vi "Pre Launch Init.vi"(11 "Nested in":refnum<class "ENG Actor.lvclass">) -> (0 "error out":errorcluster, 3 "Nested out":refnum<class "ENG Actor.lvclass">)   [LabVIEW 2020, in "ENG Actor.lvlib" / "ENG Actor.lvclass"]
doc: "(<B>Filename</B>: Actor Framework.lvlib:Actor.lvclass:Pre Launch Init.vi)\n\nDefines behavior that occurs after the Launch Nested Actor method is invoked but before the actor's Actor Core method begins running.\n\nBy default, this method does nothing. A descendant class may override it to define behavior."
uses:
  ENG Actor.lvclass
  C:/Program Files (x86)/National Instruments/LabVIEW 2020/vi.lib/ActorFramework/Actor/Actor.lvclass
  ENG Actor.lvclass/ENG Actor.ctl
  <vilib>/ActorFramework/Actor/Actor.lvclass/Actor.ctl
  <vilib>/ActorFramework/Message Enqueuer/Message Enqueuer.lvclass/Message Enqueuer.ctl
  <vilib>/ActorFramework/Message Enqueuer/Init from Existing Queue.vi
  <vilib>/ActorFramework/Message Enqueuer/Enqueue.vi
  ENG Actor Messages/Init Msg/Init Msg.lvclass
  C:/Program Files (x86)/National Instruments/LabVIEW 2020/vi.lib/ActorFramework/Message/Message.lvclass
  <vilib>/ActorFramework/Message Priority Queue/Priority Enqueue.vi
  <vilib>/ActorFramework/Message Enqueuer/Message Enqueuer.lvclass
  <vilib>/ActorFramework/Actor/Actor.lvclass
  ENG Actor Messages/Update MSG Msg/Update MSG Msg.lvclass
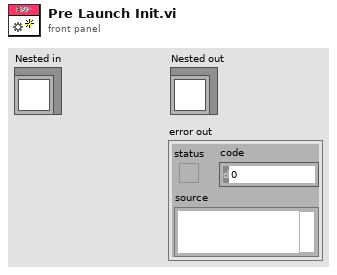
[diagram p1: front panel]
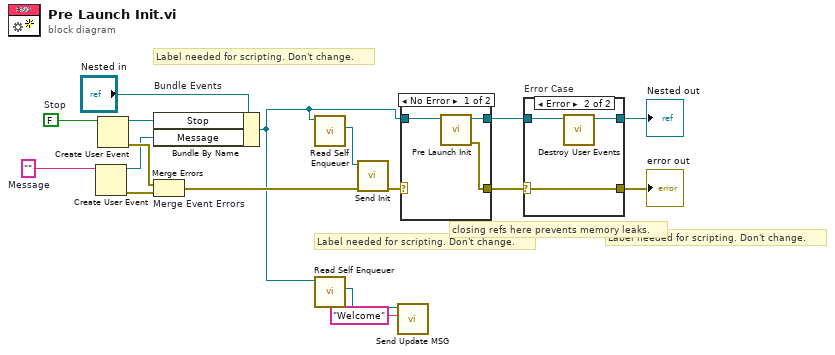
[diagram p0: block diagram]
diagram:
  w5 = ""  # Message
  w16 = FALSE  # Stop
  # "Label needed for scripting. Don't change."
  # "Label needed for scripting. Don't change."
  # "Label needed for scripting. Don't change."
  # "closing refs here prevents memory leaks."
  n1 = Create User Event(user event datatype=w5) -> (user event=w4:refnum<user-event>, error out=w3:errorcluster)  [unwired: 1 in]
  n2 = Create User Event(user event datatype=w16) -> (user event=w13:refnum<user-event>, error out=w15:errorcluster)  [unwired: 1 in]
  n3 = Bundle By Name "Bundle Events"(cluster="Nested in", "Stop"=w13, "Message"=w4) -> (w6:refnum<class "ENG Actor.lvclass">)
  n4 = Merge Errors "Merge Event Errors"(w15, w3) -> (w8:errorcluster)
  n5 = call <vilib>:"Read Self Enqueuer.vi"("Actor"=w6) -> ("Self Enqueuer"=w9:refnum<class "Message Enqueuer.lvclass">)  [unwired: 10 in]
  n6 = call <vilib>:"Read Self Enqueuer.vi"("Actor"=w6) -> ("Self Enqueuer"=w2:refnum<class "Message Enqueuer.lvclass">)  [unwired: 10 in]
  n7 = call "Send Init.vi"("error in (no error)"=w8, "Message Enqueuer"=w9) -> ("error out"=w7:errorcluster)  [unwired: 8 in, 1 out]
  n8 = call "Send Update MSG.vi"("Update MSG"="Welcome", "Message Enqueuer"=w2) -> ()  [unwired: 8 in, 2 out]
  n9 = case shown="No Error" w7 {
    selector: w7 -> [_ w22]
    tunnel: [w20 w21] -> w11
    tunnel: w6 -> [w19 w21]
    tunnel: [w18 w22] -> w10
    frame No Error {
      n10 = call-parent "Pre Launch Init.vi"("Actor in"=w19) -> ("error out"=w18:errorcluster, "Actor out"=w20:refnum<class "ENG Actor.lvclass">)  [unwired: 9 in]
    }
    frame Error {
    }
  }
  n11 = case "Error Case" shown="Error" w10 {
    selector: w10 -> [w23 w27]
    tunnel: w11 -> [w24 w26]
    tunnel: [w24 w25] -> w14
    tunnel: [w23 w27] -> w12
    frame No Error {
    }
    frame Error {
      n12 = call "Destroy User Events.vi"("UI Template in"=w26) -> ("UI Template out"=w25:refnum<class "ENG Actor.lvclass">)  [unwired: 10 in]
    }
  }
  "error out" <- w12
  "Nested out" <- w14
